vi "picoquant_aux_loop.vi"(8 "error in (no error)":errorcluster, 9 "panel_in":refnum<class "panel.lvclass">, 10 "ui_user_events":T1, 11 "picoquant_generic in":refnum<class "picoquant_generic.lvclass">) -> (0 "error out":errorcluster, 1 "panel_out":refnum<class "panel.lvclass">, 3 "picoquant_generic out":refnum<class "picoquant_generic.lvclass">)   [LabVIEW 2015, in "picoquant_generic.lvclass"]
uses:
  picoquant_generic.lvclass
  UI/front_panel_class/ui_user_events.ctl
  UI/panel_class/panel.lvclass
  picoquant_generic.lvclass/picoquant_generic.ctl
  loop_notifier_tdef.ctl
panel:
  in  "stop":bool
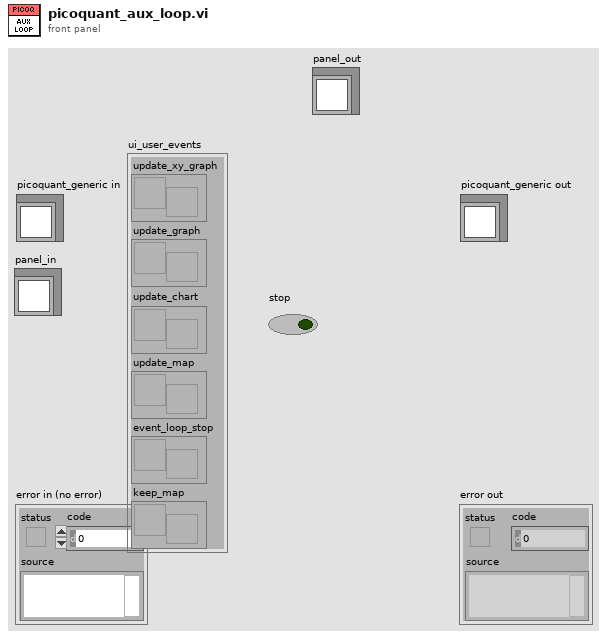
[diagram p1: front panel]
types:
  T1 = typedef "ui_user_events.ctl" = cluster{"update_xy_graph":refnum<user-event>, "update_graph":refnum<user-event>, "update_chart":refnum<user-event>, "update_map":refnum<user-event>, "event_loop_stop":refnum<user-event>, "keep_map":refnum<user-event>}
  T2 = typedef "loop_notifier_tdef.ctl" = enum16{"exit"}
  T3 = typedef "hydraharp_count_rates.ctl" = cluster{"channel_rates":i32[], "sync_rate":i32}
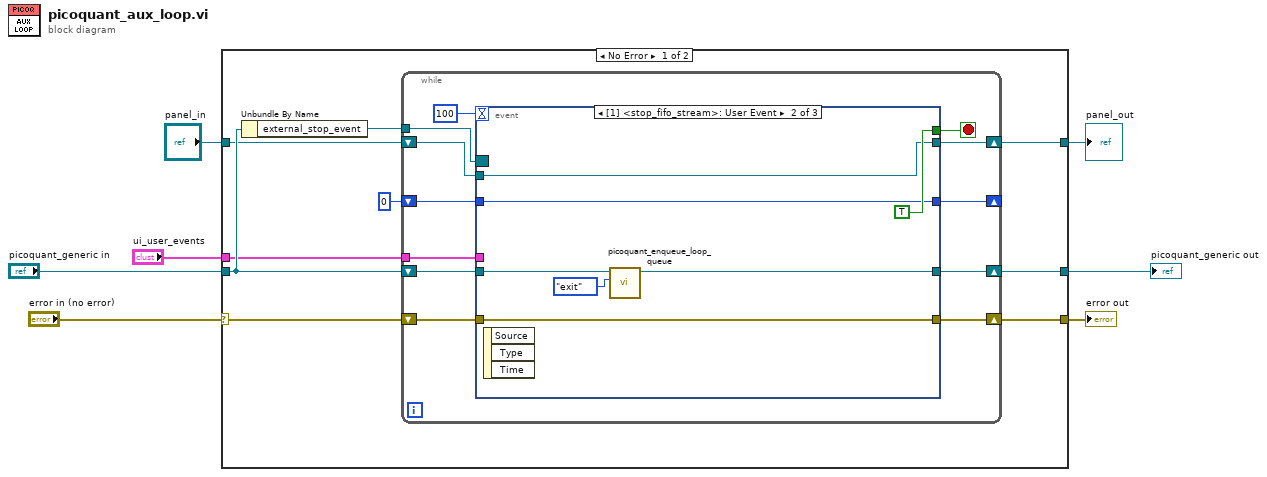
[diagram p0: block diagram]
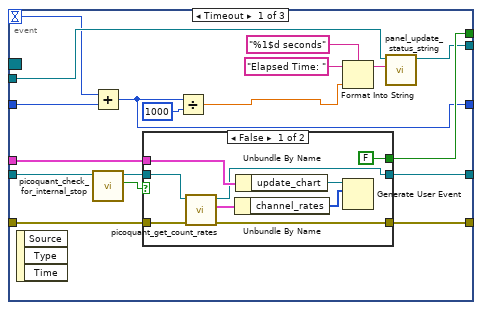
[diagram p2: hidden frame]
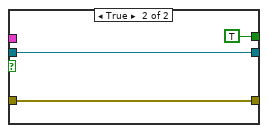
[diagram p3: hidden frame]
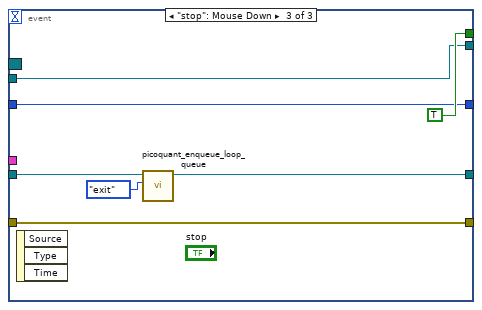
[diagram p4: hidden frame]
diagram:
  n1 = case shown="No Error" "error in (no error)" {
    selector: "error in (no error)" -> [w13 w75]
    tunnel: [w11 w75] -> w6
    tunnel: [w15 w74] -> w4
    tunnel: "picoquant_generic in" -> [w16 w74]
    tunnel: "ui_user_events" -> [w14 _]
    tunnel: "panel_in" -> [w10 w73]
    tunnel: [w9 w73] -> w1
    frame No Error {
      n2 = Unbundle By Name(w16) -> ("external_stop_event"=w12:refnum<event-registration>)
      n3 = while {
        tunnel: w12 -> [w28]
        shift-right: [w25] -> w15
        shift-left: w16 -> [w26]
        tunnel: w14 -> [w23]
        shift-right: [w21] -> w11
        shift-left: w13 -> [w22]
        shift-right: [w19] -> w9
        shift-left: w10 -> [w20]
        shift-right: [w17] -> _
        shift-left: 0 -> [w18]
        stop <- w27 stop-if-true
        n4 = event shown="[1] <stop_fifo_stream>: User Event" {
          selector: w28 -> [_ _ _]
          dyn-events: _ -> [_ _ _]
          timeout: 100 -> [w33 _ _]
          tunnel: [w46 TRUE TRUE] -> w27
          tunnel: w26 -> [w40 w64 w69]
          tunnel: [w44 w62 w68] -> w25
          tunnel: w23 -> [w45 _ _]
          tunnel: w22 -> [w42 w60 w71]
          tunnel: [w43 w60 w71] -> w21
          tunnel: w20 -> [w38 w61 w67]
          tunnel: [w37 w61 w67] -> w19
          tunnel: w18 -> [w32 w59 w66]
          tunnel: [w30 w59 w66] -> w17
          event Timeout {
            n5 = event-data() -> ()  [unwired: 1 in, 3 out]
            n6 = Add(x=w33, y=w32) -> (x+y=w30:i32)
            n7 = call "picoquant_check_for_internal_stop.vi"("picoquant_generic in"=w40) -> ("exit?"=w41:bool, "picoquant_generic out"=w39:refnum<class "picoquant_generic.lvclass">)  [unwired: 8 in, 1 out]
            n8 = case shown="False" w41 {
              tunnel: [FALSE TRUE] -> w46
              tunnel: w45 -> [w54 _]
              tunnel: w39 -> [w52 w57]
              tunnel: [w49 w57] -> w44
              tunnel: [w47 w58] -> w43
              tunnel: w42 -> [w48 w58]
              frame False {
                n9 = call-dynamic "picoquant_get_count_rates.vi"("error in (no error)"=w48, "picoquant_generic in"=w52) -> ("error out"=w47:errorcluster, "count_rates"=w51:T3, "picoquant_generic out"=w49:refnum<class "picoquant_generic.lvclass">)  [unwired: 7 in]
                n10 = Unbundle By Name(w51) -> ("channel_rates"=w50:i32[])
                n11 = Unbundle By Name(w54) -> ("update_chart"=w53:refnum<user-event>)
                n12 = Generate User Event(user event=w53, event data cluster=w50) -> ()  [unwired: 2 in, 2 out]
              }
              frame True {
              }
            }
            n13 = Divide(x=w30, y=1000) -> (x/y=w29:dbl)
            n14 = Format Into String(format string="%1$d seconds", initial string="Elapsed Time: ", w29) -> (resulting string=w31:string)  [unwired: 1 in, 1 out]
            n15 = call-dynamic "panel_update_status_string.vi"("String"=w31, "panel in"=w38) -> ("panel out"=w37:refnum<class "panel.lvclass">)  [unwired: 8 in, 1 out]
          }
          event User Event {
            n16 = event-data() -> ()  [unwired: 1 in, 3 out]
            n17 = call "picoquant_enqueue_loop_queue.vi"("loop_notifier"=loop_notifier_tdef."exit" ("notification"), "picoquant_generic in"=w64) -> ("picoquant_generic out"=w62:refnum<class "picoquant_generic.lvclass">)  [unwired: 8 in, 1 out]
          }
          event "stop": Mouse Down {
            n18 = event-data() -> ()  [unwired: 1 in, 3 out]
            n19 = call "picoquant_enqueue_loop_queue.vi"("loop_notifier"=loop_notifier_tdef."exit" ("element"), "picoquant_generic in"=w69) -> ("picoquant_generic out"=w68:refnum<class "picoquant_generic.lvclass">)  [unwired: 8 in, 1 out]
          }
        }
      }
    }
    frame Error {
    }
  }
  "error out" <- w6
  "picoquant_generic out" <- w4
  "panel_out" <- w1
